vi "TMCM351-Step.vi"(4 "执行完毕":bool, 5 "错误输入":errorcluster caption="错误输入（无错误）", 6 "Step":i32, 7 "motor":u8(ring) items=["x", "y", "z"], 8 "com in":refnum<visa-resource-name>) -> (0 "错误输出":errorcluster, 3 "com out":refnum<visa-resource-name>)   [LabVIEW 2018]
uses:
  module_param.vi
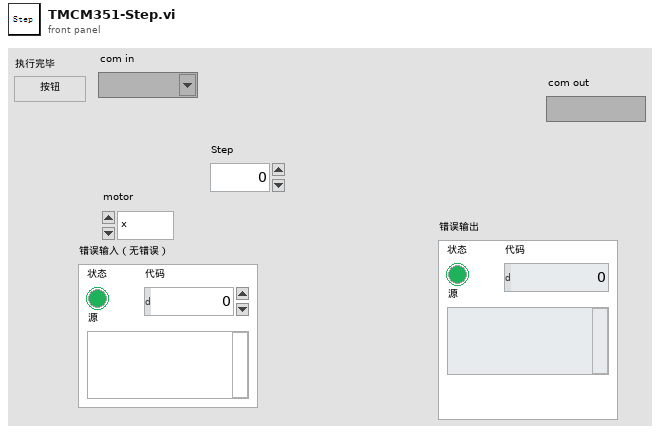
[diagram p1: front panel]
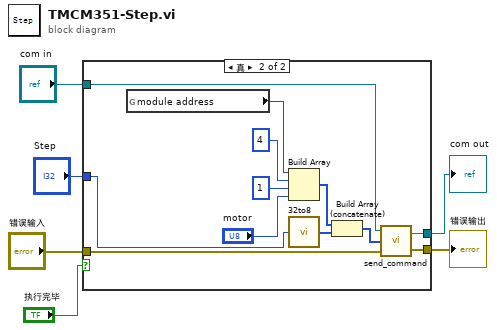
[diagram p0: block diagram]
diagram:
  n1 = case shown="真" "执行完毕" {
    tunnel: "com in" -> [w8 w13]
    tunnel: "Step" -> [_ w12]
    tunnel: [w8 w11] -> w3
    tunnel: [w7 w10] -> w2
    tunnel: "错误输入" -> [w7 w9]
    frame False {
    }
    frame True {
      n2 = global read "module_param.vi" "module address"() -> (w18:u8)
      n3 = Build Array(w18, u8 4, u8 1, "motor") -> (w16:u8[])
      n4 = call "32to8.vi"("32data_in"=w12) -> ("8Array"=w15:u8[])
      n5 = Build Array (concatenate)(w16, w15) -> (w14:u8[])
      n6 = call "send_command.vi"("错误输入"=w9, 3:w14, "com in"=w13) -> ("错误输出"=w10:errorcluster, "com out"=w11:refnum<visa-resource-name>)
    }
  }
  "com out" <- w3
  "错误输出" <- w2
